vi "Send Dispatcher Command.vi"(7 "Command":T1=enum."Rx", 8 "error in (no error)":errorcluster, 9 "timeout in ms (0)":i32 format="%d ms", 10 "Parameters":T2, 11 "Dispatcher Interface in":refnum<class "Dispatcher Interface.lvclass">) -> (0 "error out":errorcluster, 3 "Dispatcher Interface out":refnum<class "Dispatcher Interface.lvclass">)   [LabVIEW 2021, in "DSF Core.lvlib" / "Dispatcher Interface.lvclass"]
uses:
  Dispatcher Interface.lvclass
  Rx Parameters.ctl
  Command.ctl
  Parameters.ctl
  Command Data.ctl
  Write Dispatcher Command.vi
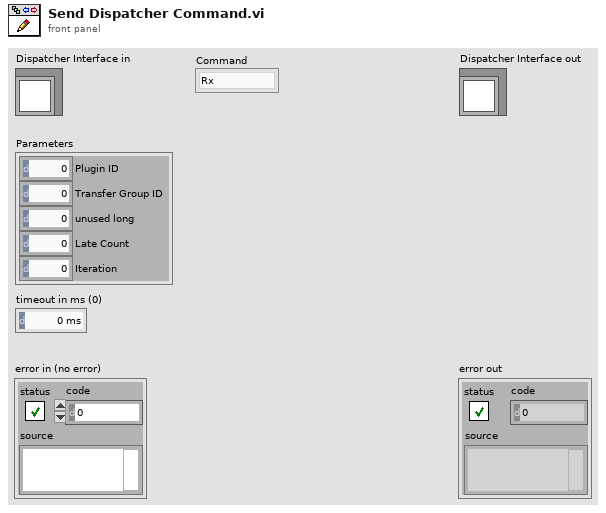
[diagram p1: front panel]
types:
  T1 = typedef "DSF Core.lvlib/Dispatcher Interface.lvclass/Command.ctl" = enum8{"Idle", "Start", "Rx", "Tx", "Set Inline Buffer", "Shutdown", "Error"}
  T2 = typedef "DSF Core.lvlib/Dispatcher Interface.lvclass/Rx Parameters.ctl" = cluster{"Plugin ID":u8, "Transfer Group ID":u8, "unused long":u16, "Late Count":i32, "Iteration":u64}
  T3 = typedef "DSF Core.lvlib/Dispatcher Interface.lvclass/Parameters.ctl" = cluster{"arg1":u64, "arg2":u64}
  T4 = typedef "DSF Core.lvlib/Dispatcher Interface.lvclass/Command Data.ctl" = cluster{"Command":T1, "Parameters":T3}
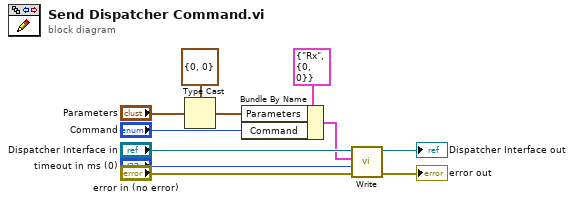
[diagram p0: block diagram]
diagram:
  n1 = Type Cast(type=T3 {"arg1"=0, "arg2"=0} ("Parameters"), x="Parameters") -> (*(type *) &x=w4:T3)
  n2 = Bundle By Name(cluster=T4 {"Command"=enum."Rx", "Parameters"={"arg1"=0, "arg2"=0}} ("command"), "Parameters"=w4, "Command"="Command") -> (w3:T4)
  n3 = call-poly "Write.vi"("error in (no error)"="error in (no error)", "timeout in ms (0)"="timeout in ms (0)", "command"=w3, "Dispatcher Interface in"="Dispatcher Interface in") -> ("error out"=→"error out":errorcluster, "Dispatcher Interface out"=→"Dispatcher Interface out":refnum<class "Dispatcher Interface.lvclass">)  [unwired: 6 in]
